vi "CreateExperimentLogColumnHeaders.vi"() -> (3 "Column Headers":string)   [LabVIEW 2012]
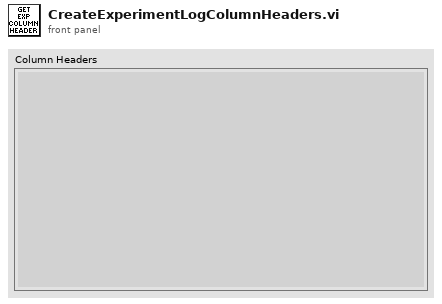
[diagram p1: front panel]
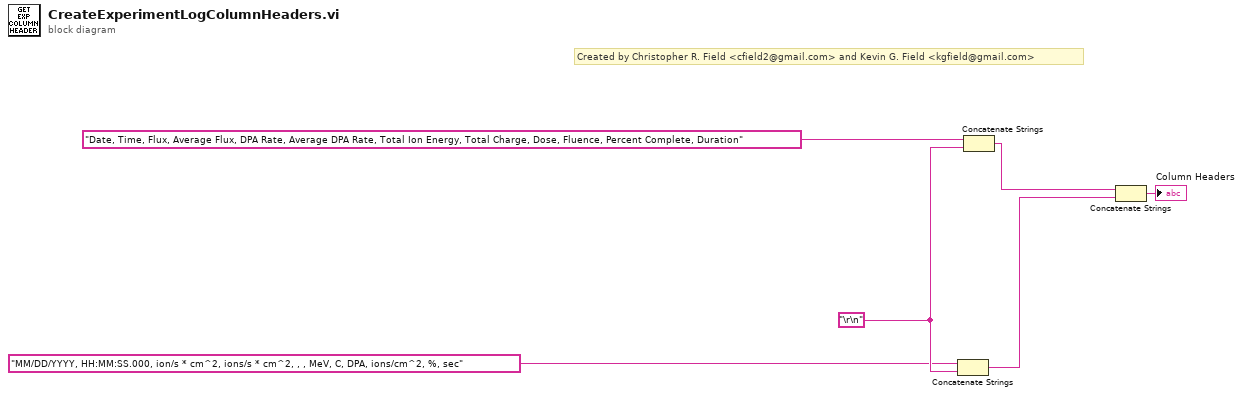
[diagram p0: block diagram]
diagram:
  w2 = "\r\n"
  # "Created by Christopher R. Field <cfield2@gmail.com> and Kevin G. Field <kgfield@gmail.com>"
  n1 = Concatenate Strings("MM/DD/YYYY, HH:MM:SS.000, ion/s * cm^2, ions/s * cm^2, , , MeV, C, DPA, ions/cm^2, %, sec", w2) -> (w4:string)
  n2 = Concatenate Strings("Date, Time, Flux, Average Flux, DPA Rate, Average DPA Rate, Total Ion Energy, Total Charge, Dose, Fluence, Percent Complete, Duration", w2) -> (w5:string)
  n3 = Concatenate Strings(w5, w4) -> (→"Column Headers":string)
